vi "createDeviceXmlElement.vi"(6 "lastcal":string, 7 "serial":string, 8 "error in (no error)":errorcluster, 9 "name":string, 10 "setup ref":refnum<k20>, 11 "DOM document":refnum<k20>) -> (0 "error out":errorcluster, 2 "dup setup ref":refnum<k20>, 3 "dup DOM document":refnum<k20>)   [LabVIEW 2013, in "XML.lvlib"]
uses:
  <vilib>/xml/Close Reference(Node).vi
  lib/XML.lvlib
  <resource>/objmgr/DOMUserDefRef.rc
  <vilib>/xml/NI_XML.lvlib
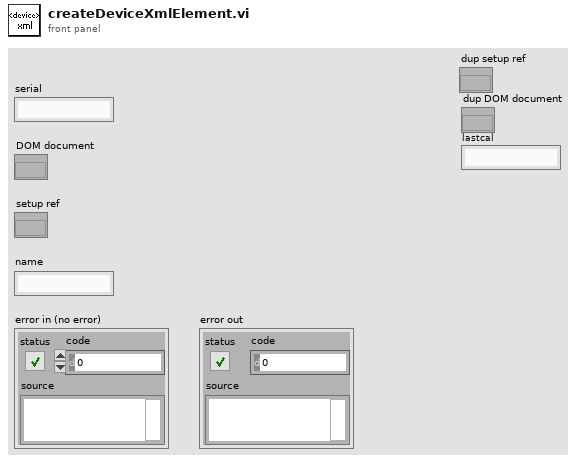
[diagram p1: front panel]
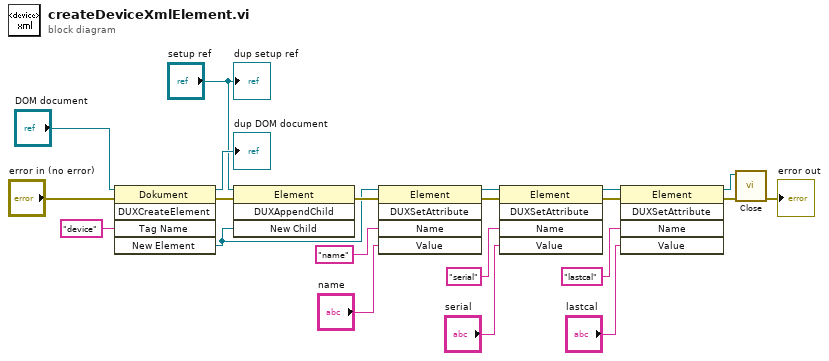
[diagram p0: block diagram]
diagram:
  n1 = invoke class="Dokument" method="DUXCreateElement"(reference="DOM document", error in="error in (no error)", "Tag Name"="device") -> (reference out=→"dup DOM document":refnum<k20>, error out=w12:errorcluster, "New Element"=w8:refnum<k20>)  [unwired: 2 in, 2 out]
  n2 = invoke class="Element" method="DUXAppendChild"(reference="setup ref", error in=w12, "New Child"=w8) -> (error out=w14:errorcluster)  [unwired: 1 in, 3 out]
  n3 = invoke class="Element" method="DUXSetAttribute"(reference=w8, error in=w14, "Name"="name", "Value"="name") -> (reference out=w17:refnum<k20>, error out=w18:errorcluster)  [unwired: 1 in, 3 out]
  n4 = invoke class="Element" method="DUXSetAttribute"(reference=w17, error in=w18, "Name"="serial", "Value"="serial") -> (reference out=w6:refnum<k20>, error out=w5:errorcluster)  [unwired: 1 in, 3 out]
  n5 = invoke class="Element" method="DUXSetAttribute"(reference=w6, error in=w5, "Name"="lastcal", "Value"="lastcal") -> (reference out=w3:refnum<k20>, error out=w4:errorcluster)  [unwired: 1 in, 3 out]
  n6 = call-poly <vilib>:"Close.vi"("error in (no error)"=w4, "node"=w3) -> ("error out"=→"error out":errorcluster)  [unwired: 7 out]
  "dup setup ref" <- "setup ref"
